vi "Set Test Params.vi"() -> ()   [LabVIEW 2025]
uses:
  19052 Example/controls/Step--numeric.ctl
panel:
  out "Instrument Info":string[](array[string])
  in  "IR Parameters":T1={"Voltage Level [V]"=500, "Hi Limit [ohm]"=30000000000.0, "Test Time [s] "=1.3, "Dwell Time [s]"=4.4, "Lo Limit [ohm]"=2500000.0, "Ramp Time [s] "=1.1, "Fall Time [s]"=2.2} {"Voltage Level [V]" max=6000 format="%.3p"; "Hi Limit [ohm]" format="%#_6p"; "Lo Limit [ohm]" format="%#_6p"}
  in  "DC Parameters":T2={"Voltage Level [V]"=1000, "Hi Limit [A]"=0.005, "Test Time [s] "=2.3, "Dwell Time [s]"=4.4, "Lo Limit [A]"=0.001, "ARC Limit [A]"=0.005, "Ramp Time [s] "=1.1, "Fall Time [s]"=2.2} {"Voltage Level [V]" format="%.3p"; "Hi Limit [A]" format="%#_6p"; "Lo Limit [A]" format="%#_6p"; "ARC Limit [A]" format="%#_6p"}
  in  "AC Parameters":T3={"Voltage Level [V]"=1250, "Hi Limit [A]"=0.01, "Test Time [s] "=3.3, "Lo Limit [A]"=0.001, "ARC Limit [A]"=0.007, "Ramp Time [s] "=1.1, "Fall Time [s]"=2.2} {"Voltage Level [V]" format="%.3p"; "Hi Limit [A]" format="%#_6p"; "Lo Limit [A]" format="%#_6p"; "ARC Limit [A]" format="%#_6p"}
  in  "Serial Configuration":T4={"Baud Rate"=9600, "Flow Control"=0, "Parity"=0, "Data Bits"=8, "Stop Bits"=1} {"Baud Rate" items=["300"=300, "600"=600, "1200"=1200, "2400"=2400, "4800"=4800, "9600"=9600, "19200"=19200]; "Flow Control" items=["NONE", "SOFTWARE"]; "Parity" items=["NONE", "ODD", "EVEN"]; "Data Bits" items=["7"=7, "8"=8]; "Stop Bits" items=["1"=1]}
  in  "VISA resource name":refnum<visa-resource-name>="Hi-Pot_COM6"
  # "Step 1"
  # "Step 2"
  # "Step 3"
  # "19052 SET TEST \nPARAMETERS"
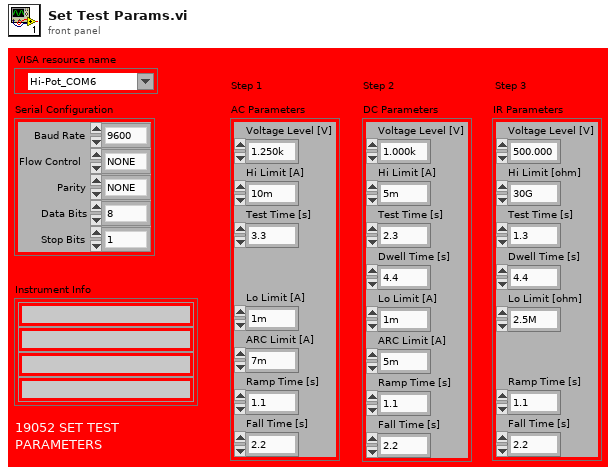
[diagram p1: front panel]
types:
  T1 = cluster{"Voltage Level [V]":u16, "Hi Limit [ohm]":dbl, "Test Time [s] ":dbl, "Dwell Time [s]":dbl, "Lo Limit [ohm]":dbl, "Ramp Time [s] ":dbl, "Fall Time [s]":dbl}
  T2 = cluster{"Voltage Level [V]":u16, "Hi Limit [A]":dbl, "Test Time [s] ":dbl, "Dwell Time [s]":dbl, "Lo Limit [A]":dbl, "ARC Limit [A]":dbl, "Ramp Time [s] ":dbl, "Fall Time [s]":dbl}
  T3 = cluster{"Voltage Level [V]":u16, "Hi Limit [A]":dbl, "Test Time [s] ":dbl, "Lo Limit [A]":dbl, "ARC Limit [A]":dbl, "Ramp Time [s] ":dbl, "Fall Time [s]":dbl}
  T4 = cluster{"Baud Rate":u32, "Flow Control":u16, "Parity":u16, "Data Bits":u16, "Stop Bits":u16}
  T5 = typedef "Step--numeric.ctl" = u8
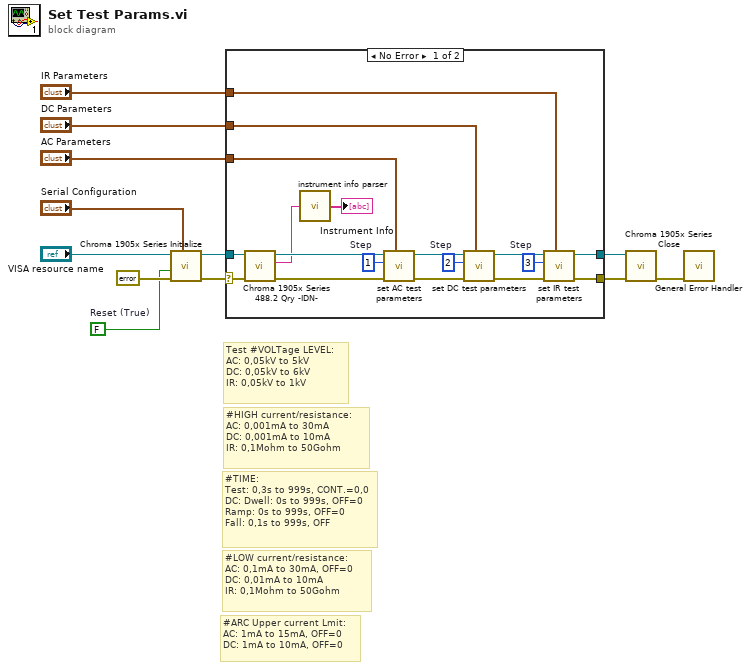
[diagram p0: block diagram]
diagram:
  w1 = FALSE  # Reset (True)
  # "#ARC Upper current Lmit:\nAC: 1mA to 15mA, OFF=0\nDC: 1mA to 10mA, OFF=0"
  # "#TIME: \nTest: 0,3s to 999s, CONT.=0,0\nDC: Dwell: 0s to 999s, OFF=0\nRamp: 0s to 999s, OFF=0\nFall: 0,1s to 999s, OFF"
  # "#LOW current/resistance: \nAC: 0,1mA to 30mA, OFF=0\nDC: 0,01mA to 10mA\nIR: 0,1Mohm to 50Gohm"
  # "#HIGH current/resistance: \nAC: 0,001mA to 30mA\nDC: 0,001mA to 10mA\nIR: 0,1Mohm to 50Gohm"
  # "Test #VOLTage LEVEL: \nAC: 0,05kV to 5kV\nDC: 0,05kV to 6kV\nIR: 0,05kV to 1kV"
  n1 = call "Chroma 1905x Series Initialize.vi"("Serial Configuration"="Serial Configuration", "error in (no error)"=errorcluster {"status"=FALSE, "code"=0, "source"=""}, "Reset (True)"=w1, "VISA resource name"="VISA resource name") -> ("error out"=w2:errorcluster, "VISA resource name out"=w8:refnum<visa-resource-name>)  [unwired: 6 in]
  n2 = case shown="No Error" w2 {
    selector: w2 -> [w18 w32]
    tunnel: w8 -> [w17 w31]
    tunnel: [w25 w32] -> w7
    tunnel: [w24 w31] -> w6
    tunnel: "AC Parameters" -> [w21 _]
    tunnel: "DC Parameters" -> [w20 _]
    tunnel: "IR Parameters" -> [w19 _]
    frame No Error {
      w22 = T5 2  # Step
      w23 = T5 3  # Step
      w28 = T5 1  # Step
      n3 = call "Chroma 1905x Series 488.2 Qry -IDN-.vi"("error in (no error)"=w18, "VISA resource name"=w17) -> ("error out"=w15:errorcluster, "Result"=w14:string, "VISA resource name out"=w16:refnum<visa-resource-name>)  [unwired: 7 in]
      n4 = call "instrument info parser.vi"("ID"=w14) -> ("Instrument Info"=→"Instrument Info":string[])  [unwired: 4 in]
      n5 = call "set AC test parameters.vi"("AC Parameters"=w21, "error in (no error)"=w15, "Step"=w28, "VISA Refnum in"=w16) -> ("error out"=w30:errorcluster, "VISA Refnum out"=w29:refnum<visa-resource-name>)  [unwired: 6 in]
      n6 = call "set DC test parameters.vi"("DC Parameters"=w20, "error in (no error)"=w30, "Step"=w22, "VISA Refnum in"=w29) -> ("error out"=w26:errorcluster, "VISA Refnum out"=w27:refnum<visa-resource-name>)  [unwired: 6 in]
      n7 = call "set IR test parameters.vi"("IR Parameters"=w19, "error in (no error)"=w26, "Step"=w23, "VISA Refnum in"=w27) -> ("error out"=w25:errorcluster, "VISA Refnum out"=w24:refnum<visa-resource-name>)  [unwired: 6 in]
    }
    frame Error {
    }
  }
  n8 = call "Chroma 1905x Series Close.VI"("error in (no error)"=w7, "VISA resource name"=w6) -> ("error out"=w9:errorcluster)  [unwired: 9 in]
  n9 = call <vilib>:"General Error Handler.vi"("error in (no error)"=w9) -> ()  [unwired: 10 in, 5 out]
